vi "Oscillate.vi"(0 "controller in":refnum<k24>, 1 "Cycles":i32, 2 "NumFreqs":i32, 5 "Distance":dbl, 7 "Frequency":dbl, 9 "axis name":string, 11 "error in (no error)":errorcluster, 12 "executeInBgThread":bool) -> (4 "controller out":refnum<k24>, 15 "error out":errorcluster)   [LabVIEW 2010]
uses:
  c:/aerotech/controller/5.xx.xxx/ensemble/pc/labview/2010/bin/Aerotech.Ensemble.dll
  bin/Aerotech.Ensemble.dll
  c:/aerotech/controller/5.xx.xxx/ensemble/pc/labview/2010/bin/Aerotech.Ensemble.LabVIEW.dll
  bin/Aerotech.Ensemble.LabVIEW.dll
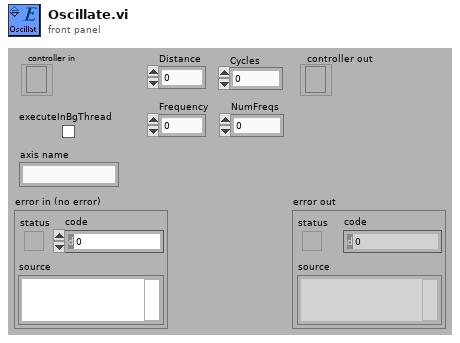
[diagram p1: front panel]
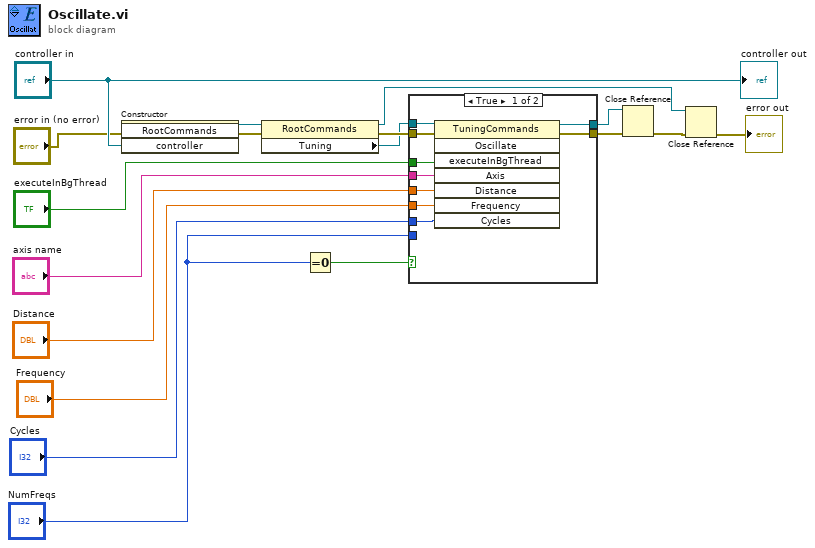
[diagram p0: block diagram]
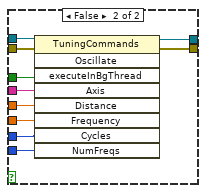
[diagram p2: hidden frame]
diagram:
  n1 = constructor class="RootCommands"(error in="error in (no error)", "controller"="controller in") -> (reference out=w7:refnum<k24>, error out=w8:errorcluster)  [unwired: 2 in, 2 out]
  n2 = property class="RootCommands"(reference=w7, error in=w8) -> (reference out=w12:refnum<k24>, error out=w6:errorcluster, "Tuning"=w5:refnum<k24>)
  n3 = Equal To 0?(x="NumFreqs") -> (x = 0?=w1:bool)
  n4 = case shown="True" w1 {
    tunnel: [w27 w35] -> w10
    tunnel: [w26 w34] -> w9
    tunnel: w6 -> [w25 w37]
    tunnel: w5 -> [w24 w36]
    tunnel: "NumFreqs" -> [_ w33]
    tunnel: "axis name" -> [w23 w31]
    tunnel: "Distance" -> [w22 w32]
    tunnel: "executeInBgThread" -> [w21 w30]
    tunnel: "Frequency" -> [w19 w29]
    tunnel: "Cycles" -> [w20 w28]
    frame True {
      n5 = invoke class="TuningCommands" method="Oscillate"(reference=w24, error in=w25, "executeInBgThread"=w21, "Axis"=w23, "Distance"=w22, "Frequency"=w19, "Cycles"=w20) -> (reference out=w27:refnum<k24>, error out=w26:errorcluster)  [unwired: 1 in, 6 out]
    }
    frame False {
      n6 = invoke class="TuningCommands" method="Oscillate"(reference=w36, error in=w37, "executeInBgThread"=w30, "Axis"=w31, "Distance"=w32, "Frequency"=w29, "Cycles"=w28, "NumFreqs"=w33) -> (reference out=w35:refnum<k24>, error out=w34:errorcluster)  [unwired: 1 in, 7 out]
    }
  }
  n7 = Close Reference(reference=w10, error in (no error)=w9) -> (error out=w11:errorcluster)
  n8 = Close Reference(reference=w12, error in (no error)=w11) -> (error out=→"error out":errorcluster)
  "controller out" <- "controller in"
